vi "Get 1 Object.vi"(8 "error in":errorcluster, 10 "instrument object":refnum<class "Abstract_Instrument.lvclass">[](array[class]), 11 "pin_name":string) -> (0 "error out":errorcluster, 3 "function object":refnum<class "Measure_Voltage.lvclass">)   [LabVIEW 2021, in "Measure_Voltage.lvclass"]
uses:
  Measure_Voltage.lvclass
  Instruments/Abstract_Instrument/Abstract_Instrument.lvclass
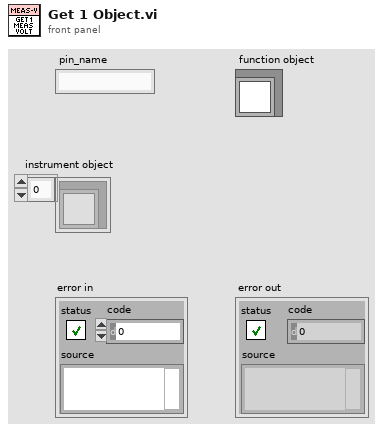
[diagram p1: front panel]
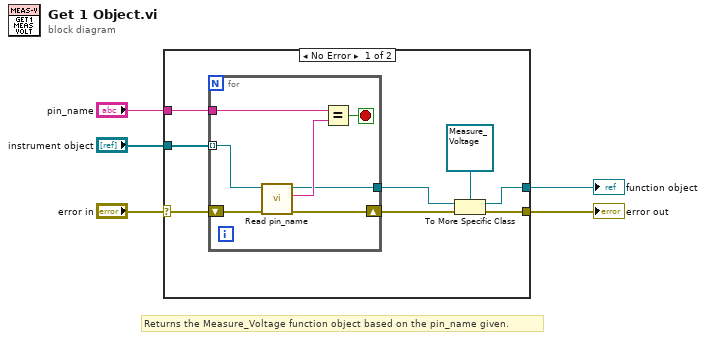
[diagram p0: block diagram]
diagram:
  # "Returns the Measure_Voltage function object based on the pin_name given."
  n1 = case shown="No Error" "error in" {
    selector: "error in" -> [w10 w21]
    tunnel: [w13 w21] -> w5
    tunnel: [w11 _] -> w4
    tunnel: "instrument object" -> [w8 _]
    tunnel: "pin_name" -> [w7 _]
    frame No Error {
      n2 = for {
        shift-right: [w19] -> w9
        shift-left: w10 -> [w20]
        tunnel: w8 -> [w18] mode=indexing
        tunnel: w7 -> [w16]
        tunnel: [w14] -> w6
        stop <- w15 stop-if-true
        n3 = call-dynamic "Read pin_name.vi"("error in (no error)"=w20, "Abstract_Instrument in"=w18) -> ("error out"=w19:errorcluster, "pin_name"=w17:string, "Abstract_Instrument out"=w14:refnum<class "Abstract_Instrument.lvclass">)  [unwired: 7 in]
        n4 = Equal?(x=w16, y=w17) -> (x = y?=w15:bool)
      }
      n5 = To More Specific Class(target class=refnum<class "Measure_Voltage.lvclass"> refnum ("Measure_Voltage.lvclass"), reference=w6, error in=w9) -> (specific class reference=w11:refnum<class "Measure_Voltage.lvclass">, error out=w13:errorcluster)
    }
    frame Error {
    }
  }
  "error out" <- w5
  "function object" <- w4
